vi "Avg ILC Data.vi"(8 "error in (no error)":errorcluster, 9 "Before This Time":dbl, 10 "After This Time":dbl, 11 "Model in":refnum<class "Model.lvclass">) -> (0 "error out":errorcluster, 2 "Force":dbl, 3 "Model out":refnum<class "Model.lvclass">)   [LabVIEW 2016, in "Model.lvclass"]
uses:
  Model.lvclass
  Model.lvclass/Model.ctl
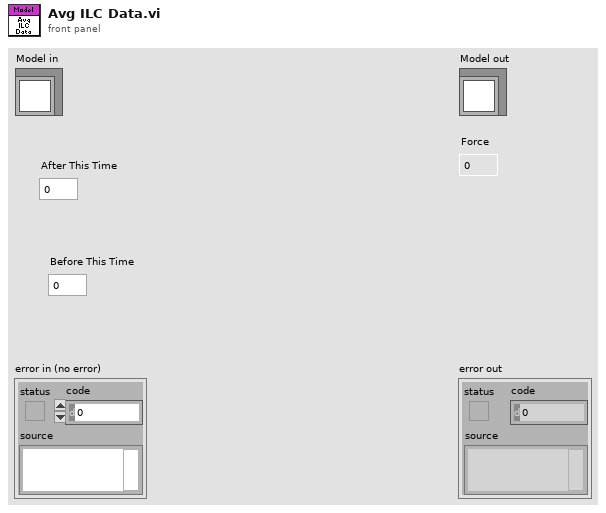
[diagram p1: front panel]
types:
  T1 = typedef "ActuatorData.ctl" = cluster{"Timestamp":dbl, "Force":dbl, "Encoder Value":i32}
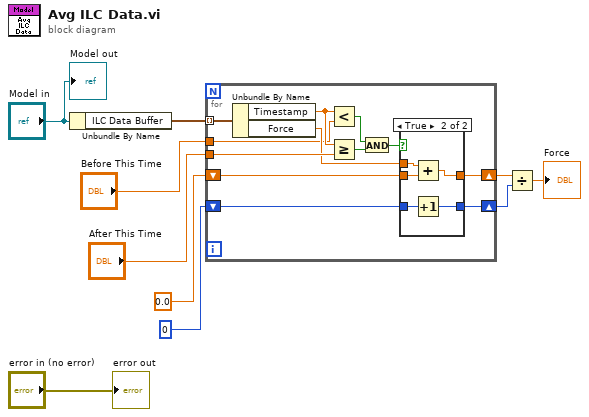
[diagram p0: block diagram]
diagram:
  n1 = Unbundle By Name("Model in") -> ("ILC Data Buffer"=w10:T1[])
  n2 = for {
    tunnel: w10 -> [w22] mode=indexing
    tunnel: "After This Time" -> [w21]
    shift-right: [w19] -> w6
    shift-left: 0.0 -> [w18]
    shift-right: [w16] -> w5
    shift-left: 0 -> [w17]
    tunnel: "Before This Time" -> [w14]
    n3 = Unbundle By Name(w22) -> ("Timestamp"=w15:dbl, "Force"=w20:dbl)
    n4 = Less?(x=w15, y=w14) -> (x < y?=w13:bool)
    n5 = Greater Or Equal?(x=w15, y=w21) -> (x >= y?=w12:bool)
    n6 = And(x=w13, y=w12) -> (x .and. y?=w11:bool)
    n7 = case shown="True" w11 {
      tunnel: w20 -> [_ w29]
      tunnel: [w23 w28] -> w19
      tunnel: w18 -> [w23 w27]
      tunnel: w17 -> [w24 w26]
      tunnel: [w24 w25] -> w16
      frame False {
      }
      frame True {
        n8 = Add(x=w29, y=w27) -> (x+y=w28:dbl)
        n9 = Increment(x=w26) -> (x+1=w25:i32)
      }
    }
  }
  n10 = Divide(x=w6, y=w5) -> (x/y=→"Force":dbl)
  "error out" <- "error in (no error)"
  "Model out" <- "Model in"
